vi "BreakStrByLenFront.vi"(8 "error in":errorcluster caption="错误输入", 9 "Front":string="AG TRG", 10 "Index":u32, 11 "StrIn":string) -> (0 "error out":errorcluster caption="错误输出", 3 "ArrayOut":string[](array[string]))   [LabVIEW 2013]
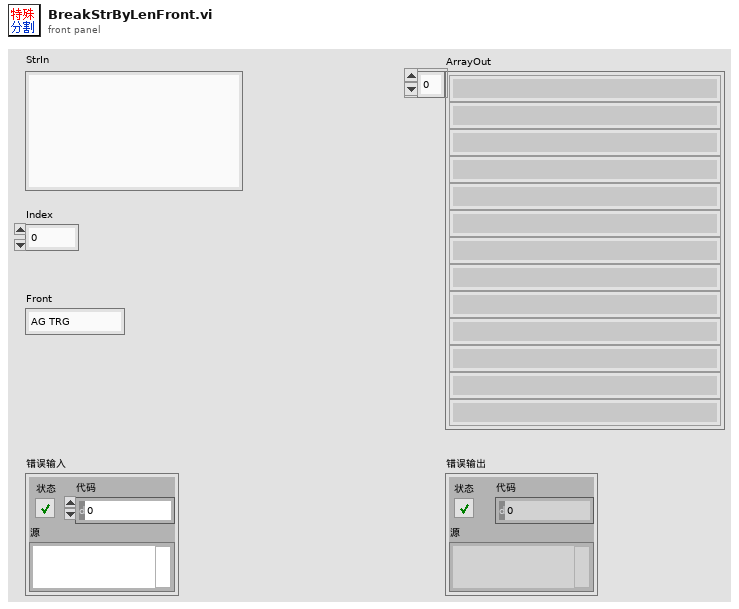
[diagram p1: front panel]
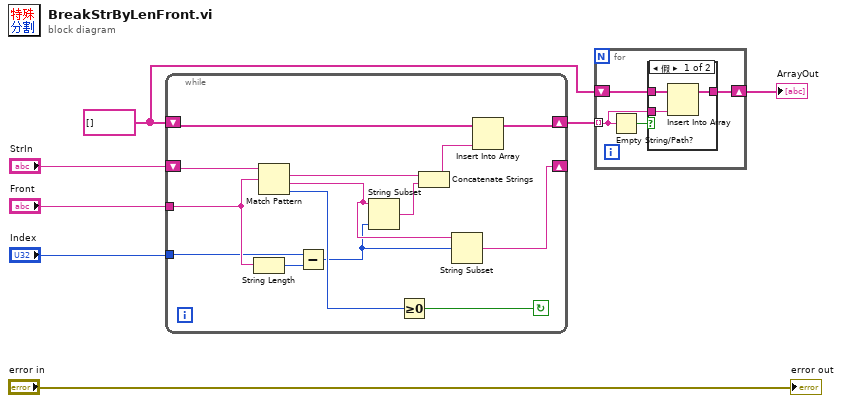
[diagram p0: block diagram]
diagram:
  w3 = string[] []
  n1 = while {
    tunnel: "Index" -> [w16]
    tunnel: "Front" -> [w17]
    shift-right: [w12] -> w4
    shift-left: w3 -> [w13]
    shift-right: [w8] -> _
    shift-left: "StrIn" -> [w21]
    stop <- w19 continue-if-true
    n2 = String Length(string=w17) -> (length=w15:i32)
    n3 = Match Pattern(string=w21, regular expression=w17) -> (match substring=w18:string, after substring=w10:string, offset past match=w20:i32)  [unwired: 1 in, 1 out]
    n4 = Subtract(x=w16, y=w15) -> (x-y=w9:u32)
    n5 = String Subset(string=w10, length (rest)=w9) -> (substring=w11:string)  [unwired: 1 in]
    n6 = Greater Or Equal To 0?(x=w20) -> (x >= 0?=w19:bool)
    n7 = Concatenate Strings(w18, w11) -> (w14:string)
    n8 = String Subset(string=w10, offset (0)=w9) -> (substring=w8:string)  [unwired: 1 in]
    n9 = Insert Into Array(array=w13, new element=w14) -> (w12:string[])  [unwired: 1 in]
  }
  n10 = for {
    tunnel: w4 -> [w23] mode=indexing
    shift-right: [w22] -> w2
    shift-left: w3 -> [w24]
    n11 = Empty String/Path?(string/path=w23) -> (empty?=w25:bool)
    n12 = case shown="假" w25 {
      tunnel: w24 -> [w28 w29]
      tunnel: w23 -> [w27 _]
      tunnel: [w26 w29] -> w22
      frame False {
        n13 = Insert Into Array(array=w28, new element=w27) -> (w26:string[])  [unwired: 1 in]
      }
      frame True {
      }
    }
  }
  "ArrayOut" <- w2
  "error out" <- "error in"
